vi "MultiTool-Track-Generate-ndipolarisFileOutput-Q-vectors-Accepts Joystick Command with Time Display-Improved PC clock in tcp loop.vi"() -> ()   [LabVIEW 2013]
panel:
  out "TIME":string
  out "bytes written":i32
  out "Return time string":string
  out "Length":u8
  out "Command":u8
  out "Tool 2":T1={"Port Handle"="", "Frame Number"=0, "Tx"=0.0, "Ty"=0.0, "Tz"=0.0, "Q0"=0.0, "Qx"=0.0, "Qy"=0.0, "Qz"=0.0, "Deviation"=0.0, " Markers Missing"=TRUE, "Out of Volume"=TRUE} {"Deviation" format="%#.4f"; "Qz" format="%#.4f"; "Qy" format="%#.4f"; "Qx" format="%#.4f"; "Q0" format="%#.4f"; "Tz" format="%#.2f"; "Ty" format="%#.2f"; "Tx" format="%#.2f"}
  in  "Location of ROM File for Tool 2":path=path "C:/Program Files (x86)/Northern Digital Inc/8700339.rom"
  in  "NDI  Running":bool=TRUE
  out "Stop Reading":bool=TRUE
  out "Start Reading":bool
  out "Object Identifier":string="0"
  in  "Track Outside Measurement Volume? (F:No)":bool
  in  "Track Stray Markers? (F:No)":bool
  out "Tool 1":T1={"Port Handle"="", "Frame Number"=0, "Tx"=0.0, "Ty"=0.0, "Tz"=0.0, "Q0"=0.0, "Qx"=0.0, "Qy"=0.0, "Qz"=0.0, "Deviation"=0.0, " Markers Missing"=TRUE, "Out of Volume"=TRUE} {"Deviation" format="%#.4f"; "Qz" format="%#.4f"; "Qy" format="%#.4f"; "Qx" format="%#.4f"; "Q0" format="%#.4f"; "Tz" format="%#.2f"; "Ty" format="%#.2f"; "Tx" format="%#.2f"}
  out "TCP loop":i32
  in  "TCP Server Running":bool=TRUE
  in  "Output Directory":path=path "C:/Users/Diogo/Desktop/NDI-Labview Gripper"
  out "NDI Loop":i32
  in  "VISA resource name":refnum<visa-resource-name>="COM8"
  in  "Reset? (T:Yes)":bool=TRUE
  in  "Location of ROM File for Tool 1":path=path "C:/Program Files (x86)/Northern Digital Inc/8700449.rom"
  in  "Serial Configuration":T2={"Baud Rate (9600)"=9600, "Flow Control (0:None)"=0, "Parity"=0, "Data Bits"=8, "Stop Bits"=10} {"Stop Bits" items=["1.0"=10, "2.0"=20]; "Parity" items=["None", "Odd", "Even"]; "Flow Control (0:None)" items=["None", "XON/XOFF"]; "Baud Rate (9600)" items=["9600"=9600, "14.4k"=14400, "19.2k"=19200, "38.4k"=38400, "57.6k "=57600, "115.2k"=115200]}
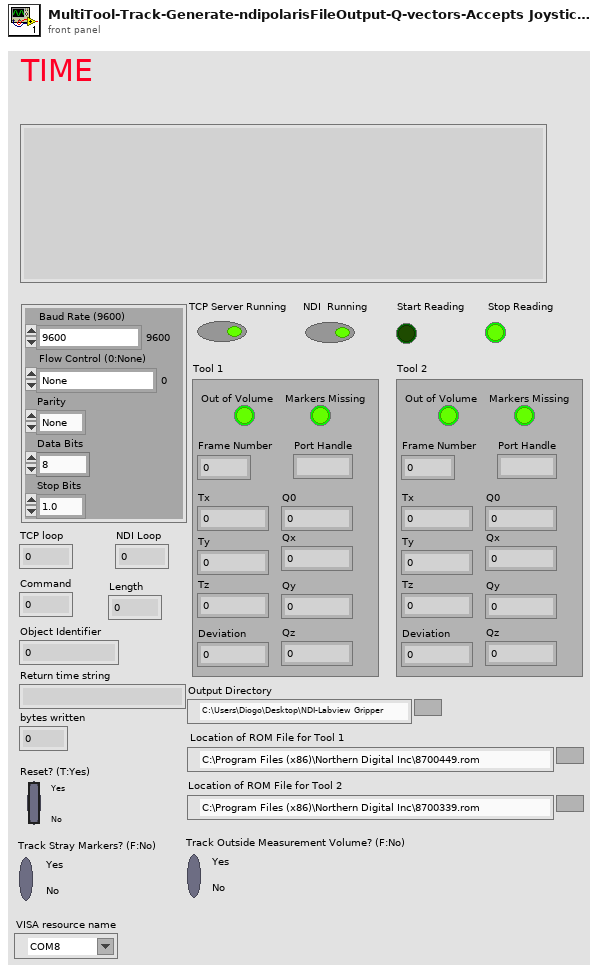
[diagram p1: front panel]
types:
  T1 = cluster{"Port Handle":string, "Frame Number":i32, "Tx":dbl, "Ty":dbl, "Tz":dbl, "Q0":dbl, "Qx":dbl, "Qy":dbl, "Qz":dbl, "Deviation":dbl, " Markers Missing":bool, "Out of Volume":bool}
  T2 = cluster{"Baud Rate (9600)":u32, "Flow Control (0:None)":u16, "Parity":u16, "Data Bits":u16, "Stop Bits":u16}
  T3 = cluster{"Port Handle":string, "Frame Number":u32, "Tx":dbl, "Ty":dbl, "Tz":dbl, "Q0":dbl, "Qx":dbl, "Qy":dbl, "Qz":dbl, "Deviation":dbl, "Missing?":bool, "Out of Volume?":bool}[]
  T4 = cluster{"Transformations[0]":cluster{"Port Handle":string, "Frame Number":u32, "Tx":dbl, "Ty":dbl, "Tz":dbl, "Q0":dbl, "Qx":dbl, "Qy":dbl, "Qz":dbl, "Deviation":dbl, "Missing?":bool, "Out of Volume?":bool}, "Transformations[1]":cluster{"Port Handle":string, "Frame Number":u32, "Tx":dbl, "Ty":dbl, "Tz":dbl, "Q0":dbl, "Qx":dbl, "Qy":dbl, "Qz":dbl, "Deviation":dbl, "Missing?":bool, "Out of Volume?":bool}, "Transformations[2]":cluster{"Port Handle":string, "Frame Number":u32, "Tx":dbl, "Ty":dbl, "Tz":dbl, "Q0":dbl, "Qx":dbl, "Qy":dbl, "Qz":dbl, "Deviation":dbl, "Missing?":bool, "Out of Volume?":bool}, "Transformations[3]":cluster{"Port Handle":string, "Frame Number":u32, "Tx":dbl, "Ty":dbl, "Tz":dbl, "Q0":dbl, "Qx":dbl, "Qy":dbl, "Qz":dbl, "Deviation":dbl, "Missing?":bool, "Out of Volume?":bool}, "Transformations[4]":cluster{"Port Handle":string, "Frame Number":u32, "Tx":dbl, "Ty":dbl, "Tz":dbl, "Q0":dbl, "Qx":dbl, "Qy":dbl, "Qz":dbl, "Deviation":dbl, "Missing?":bool, "Out of Volume?":bool}, "Transformations[5]":cluster{"Port Handle":string, "Frame Number":u32, "Tx":dbl, "Ty":dbl, "Tz":dbl, "Q0":dbl, "Qx":dbl, "Qy":dbl, "Qz":dbl, "Deviation":dbl, "Missing?":bool, "Out of Volume?":bool}, "Transformations[6]":cluster{"Port Handle":string, "Frame Number":u32, "Tx":dbl, "Ty":dbl, "Tz":dbl, "Q0":dbl, "Qx":dbl, "Qy":dbl, "Qz":dbl, "Deviation":dbl, "Missing?":bool, "Out of Volume?":bool}, "Transformations[7]":cluster{"Port Handle":string, "Frame Number":u32, "Tx":dbl, "Ty":dbl, "Tz":dbl, "Q0":dbl, "Qx":dbl, "Qy":dbl, "Qz":dbl, "Deviation":dbl, "Missing?":bool, "Out of Volume?":bool}, "Transformations[8]":cluster{"Port Handle":string, "Frame Number":u32, "Tx":dbl, "Ty":dbl, "Tz":dbl, "Q0":dbl, "Qx":dbl, "Qy":dbl, "Qz":dbl, "Deviation":dbl, "Missing?":bool, "Out of Volume?":bool}}
  T5 = cluster{"Port Handle":string, "Frame Number":u32, "Tx":dbl, "Ty":dbl, "Tz":dbl, "Q0":dbl, "Qx":dbl, "Qy":dbl, "Qz":dbl, "Deviation":dbl, "Missing?":bool, "Out of Volume?":bool}
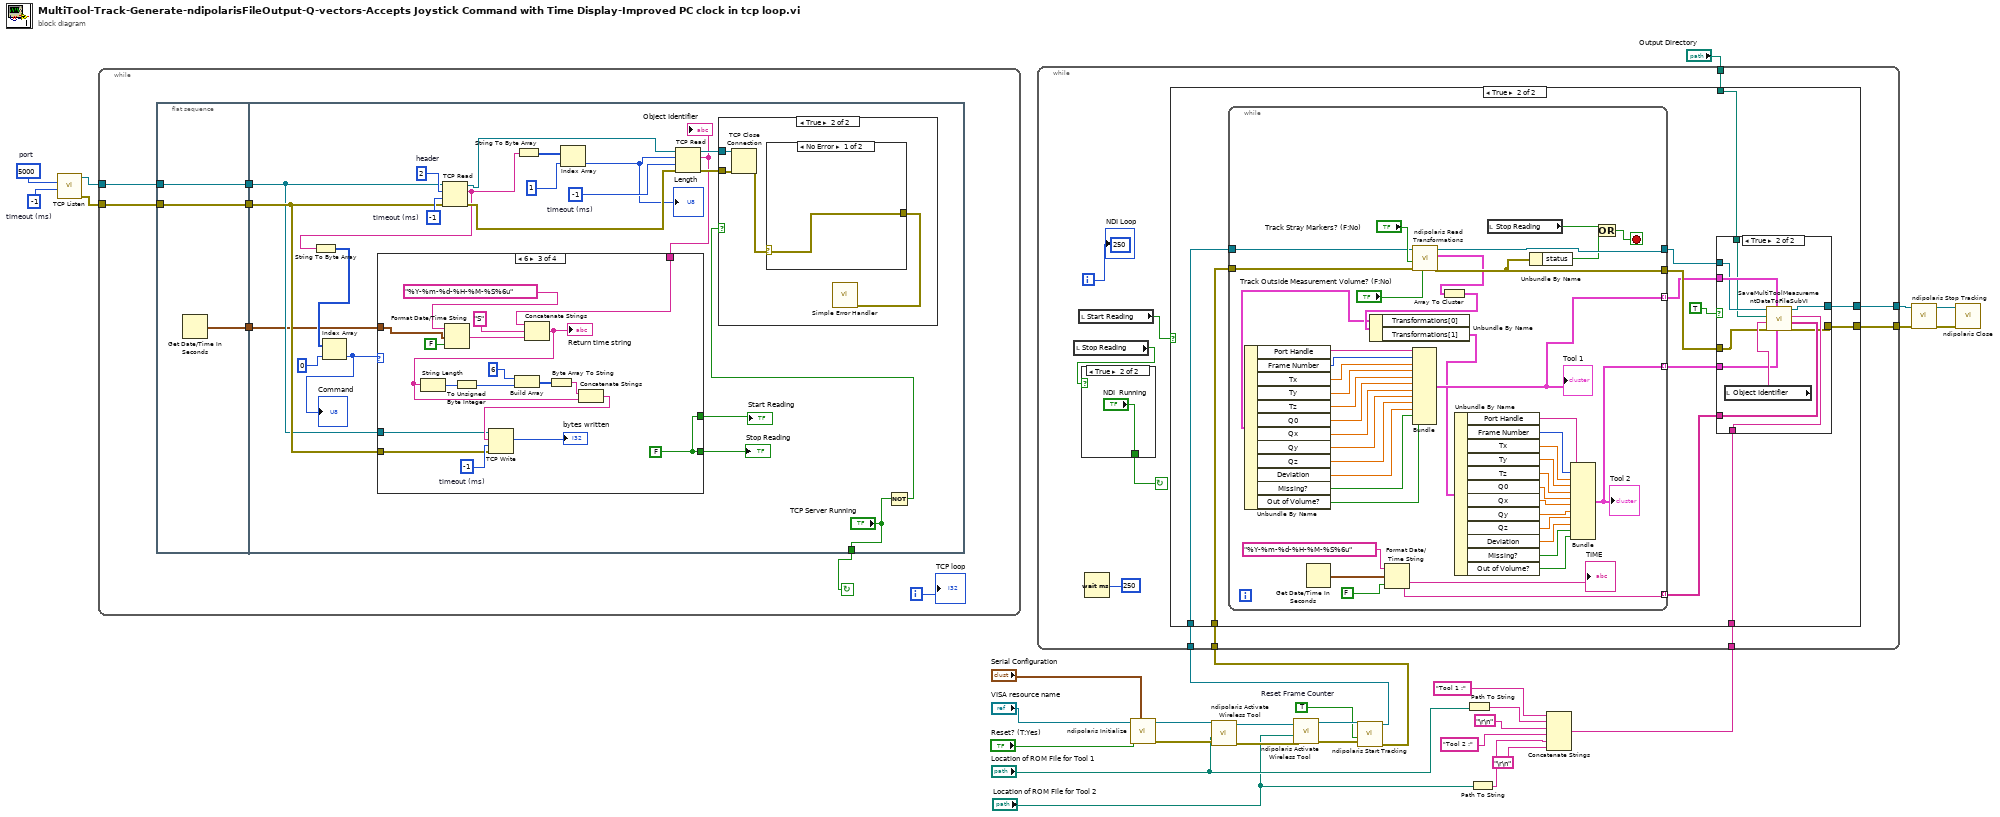
[diagram p0: block diagram]
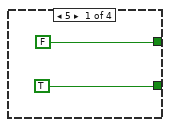
[diagram p2: hidden frame]
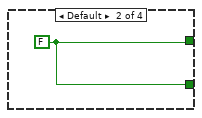
[diagram p3: hidden frame]
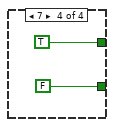
[diagram p4: hidden frame]
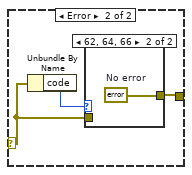
[diagram p6: hidden frame]
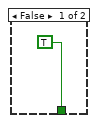
[diagram p8: hidden frame]
diagram:
  w21 = TRUE  # Reset Frame Counter
  w30 = u16 5000  # port
  w29 = i8 -1  # timeout (ms)
  n1 = call <vilib>:"TCP Listen.vi"("timeout ms (wait forever: -1)"=w29, "port"=w30) -> ("error out"=w24:errorcluster, "connection ID"=w25:refnum<k5>)  [unwired: 5 in, 3 out]
  n2 = while {
    tunnel: w25 -> [w34]
    tunnel: w24 -> [w35]
    i -> [w37]
    stop <- w36 continue-if-true
    n3 = flat-sequence {
      tunnel: w34 -> [w39]
      tunnel: w35 -> [w40]
      tunnel: [w40] -> w33
      tunnel: [w39] -> w32
      tunnel: [w38] -> w31
      tunnel: ["TCP Server Running"] -> w36
      tunnel: w33 -> [w44]
      tunnel: w32 -> [w42]
      tunnel: w31 -> [w41]
      frame #0 {
        n4 = Get Date/Time In Seconds() -> (seconds since 1Jan1904=w38:timestamp)
      }
      frame #1 {
        w58 = i8 -1  # timeout (ms)
        w61 = i8 -1  # timeout (ms)
        w62 = i8 2  # header
        n5 = TCP Read(connection ID=w42, bytes to read=w62, error in (no error)=w44, 9:w61) -> (connection ID out=w60:refnum<k5>, data out=w49:string, error out=w59:errorcluster)  [unwired: 1 in]
        n6 = String To Byte Array(string=w49) -> (unsigned byte array=w52:u8[])
        n7 = Index Array(array=w52, index=0) -> (element=w45:u8)
        "Command" <- w45
        n8 = String To Byte Array(string=w49) -> (unsigned byte array=w51:u8[])
        n9 = Index Array(array=w51, index=1) -> (element=w48:u8)
        "Length" <- w48
        n10 = TCP Read(connection ID=w60, bytes to read=w48, error in (no error)=w59, 9:w58) -> (connection ID out=w57:refnum<k5>, data out=w43:string, error out=w56:errorcluster)  [unwired: 1 in]
        "Object Identifier" <- w43
        n11 = case shown="6" w45 {
          tunnel: [FALSE w65 w67 TRUE] -> w55
          tunnel: [TRUE w65 w67 FALSE] -> w54
          tunnel: w44 -> [_ _ w70 _]
          tunnel: w43 -> [_ _ w69 _]
          tunnel: w42 -> [_ _ w68 _]
          tunnel: w41 -> [_ _ w66 _]
          frame 5 {
          }
          frame Default {
            w65 = FALSE
          }
          frame 6 {
            w79 = i8 -1  # timeout (ms)
            w67 = FALSE
            n12 = Format Date/Time String(time format string (%c)="%Y-%m-%d-%H-%M-%S%6u", seconds (now)=w66, UTC format=FALSE) -> (date/time string=w83:string)
            n13 = Concatenate Strings(w69, "S", w83) -> (w72:string)
            "Return time string" <- w72
            n14 = String Length(string=w72) -> (length=w76:i32)
            n15 = To Unsigned Byte Integer(number=w76) -> (unsigned 8bit integer=w75:u8)
            n16 = Build Array(u8 6, w75) -> (w73:u8[])
            n17 = Byte Array To String(unsigned byte array=w73) -> (string=w78:string)
            n18 = Concatenate Strings(w78, w72) -> (w71:string)
            n19 = TCP Write(connection ID=w68, data in=w71, error in (no error)=w70, 9:w79) -> (bytes written=→"bytes written":i32)  [unwired: 2 out]
          }
          frame 7 {
          }
        }
        "Start Reading" <- w55
        "Stop Reading" <- w54
        n20 = Not(x="TCP Server Running") -> (.not. x?=w46:bool)
        n21 = case shown="True" w46 {
          tunnel: w57 -> [_ w87]
          tunnel: w56 -> [_ w86]
          frame False {
          }
          frame True {
            n22 = TCP Close Connection(connection ID=w87, error in (no error)=w86) -> (error out=w88:errorcluster)  [unwired: 1 in, 1 out]
            n23 = case shown="No Error" w88 {
              selector: w88 -> [w90 w92]
              tunnel: [w90 w91] -> w89
              frame No Error {
              }
              frame Error {
                n24 = Unbundle By Name(w92) -> ("code"=w93:i32)
                n25 = case shown="62, 64, 66" w93 {
                  tunnel: w92 -> [w94 _]
                  tunnel: [w94 w95] -> w91
                  frame Default {
                  }
                  frame 62, 64, 66 {
                    w95 = errorcluster {"status"=FALSE, "code"=0, "source"=""}  # No error
                  }
                }
              }
            }
            n26 = call <vilib>:"Simple Error Handler.vi"("error in (no error)"=w89) -> ()  [unwired: 1 in, 8 out]
          }
        }
      }
    }
    "TCP loop" <- w37
  }
  n27 = call <instrlib>:"ndipolaris Initialize.vi"("Serial Configuration"="Serial Configuration", "Reset? (T: Yes)"="Reset? (T:Yes)", "VISA resource name"="VISA resource name") -> ("error out"=w11:errorcluster, "VISA resource name out"=w12:refnum<visa-resource-name>)  [unwired: 7 in]
  n28 = call <instrlib>:"ndipolaris Activate Wireless Tool.vi"("error in (no error)"=w11, "Location of ROM File for Tool"="Location of ROM File for Tool 1", "VISA resource name"=w12) -> ("error out"=w9:errorcluster, "VISA resource out"=w10:refnum<visa-resource-name>)  [unwired: 6 in, 1 out]
  n29 = call <instrlib>:"ndipolaris Activate Wireless Tool.vi"("error in (no error)"=w9, "Location of ROM File for Tool"="Location of ROM File for Tool 2", "VISA resource name"=w10) -> ("error out"=w22:errorcluster, "VISA resource out"=w23:refnum<visa-resource-name>)  [unwired: 6 in, 1 out]
  n30 = call <instrlib>:"ndipolaris Start Tracking.vi"("error in (no error)"=w22, "Reset Frame Counter? (F:No)"=w21, "VISA resource name"=w23) -> ("error out"=w16:errorcluster, "VISA resource out"=w20:refnum<visa-resource-name>)  [unwired: 7 in]
  n31 = Path To String(path="Location of ROM File for Tool 1") -> (string=w5:string)
  n32 = Path To String(path="Location of ROM File for Tool 2") -> (string=w3:string)
  n33 = Concatenate Strings("Tool 1 :" ("string"), w5, "\r\n", "Tool 2 :" ("string"), w3, "\r\n") -> (w13:string)
  n34 = while {
    tunnel: w20 -> [w105]
    tunnel: [w104] -> w17
    tunnel: w16 -> [w103]
    tunnel: "Output Directory" -> [w102]
    tunnel: [w101] -> w14
    tunnel: w13 -> [w97]
    i -> [w106]
    stop <- w96 continue-if-true
    (unwired) u8 250
    n35 = local read "Stop Reading"() -> (w98:bool)
    n36 = local read "Start Reading"() -> (w99:bool)
    n37 = case shown="True" w98 {
      tunnel: [TRUE "NDI  Running"] -> w96
      frame False {
      }
      frame True {
      }
    }
    n38 = Wait (ms)(milliseconds to wait=u32 250) -> ()  [unwired: 1 out]
    n39 = case shown="True" w99 {
      tunnel: w105 -> [w110 w122]
      tunnel: [w110 w118] -> w104
      tunnel: w103 -> [w109 w121]
      tunnel: w102 -> [_ w120]
      tunnel: [w109 w117] -> w101
      tunnel: w97 -> [_ w112]
      frame False {
      }
      frame True {
        n40 = while {
          tunnel: [w176] -> w114
          tunnel: [w175] -> w119
          tunnel: [w152] -> w115 mode=indexing
          tunnel: [w153] -> w116 mode=indexing
          tunnel: w122 -> [w151]
          tunnel: w121 -> [w150]
          tunnel: [w135] -> w111 mode=indexing
          stop <- w177 stop-if-true
          n41 = Get Date/Time In Seconds() -> (seconds since 1Jan1904=w156:timestamp)
          n42 = Format Date/Time String(time format string (%c)="%Y-%m-%d-%H-%M-%S%6u", seconds (now)=w156, UTC format=FALSE) -> (date/time string=w153:string)
          "TIME" <- w153
          n43 = call <instrlib>:"ndipolaris Read Transformations.vi"("Track Outside Measurement Volume? (F:No)"="Track Outside Measurement Volume? (F:No)", "error in (no error)"=w150, "Track Stray Markers? (F:No)"="Track Stray Markers? (F:No)", "VISA resource name"=w151) -> ("error out"=w175:errorcluster, "Transformations"=w160:T3, "VISA resource out"=w176:refnum<visa-resource-name>)  [unwired: 4 in, 1 out]
          n44 = Array To Cluster(array=w160) -> (cluster=w171:T4)
          n45 = Unbundle By Name(w171) -> ("Transformations[0]"=w170:T5, "Transformations[1]"=w148:T5)
          n46 = Unbundle By Name(w170) -> ("Port Handle"=w169:string, "Frame Number"=w168:u32, "Tx"=w167:dbl, "Ty"=w166:dbl, "Tz"=w165:dbl, "Q0"=w164:dbl, "Qx"=w163:dbl, "Qy"=w162:dbl, "Qz"=w161:dbl, "Deviation"=w159:dbl, "Missing?"=w158:bool, "Out of Volume?"=w157:bool)
          n47 = Bundle("Port Handle"=w169, "Frame Number"=w168, "Tx"=w167, "Ty"=w166, "Tz"=w165, "Q0"=w164, "Qx"=w163, "Qy"=w162, "Qz"=w161, "Deviation"=w159, "Missing?"=w158, "Out of Volume?"=w157) -> (w152:T5)  [unwired: 1 in]
          "Tool 1" <- w152
          n48 = Unbundle By Name(w148) -> ("Port Handle"=w147:string, "Frame Number"=w146:u32, "Tx"=w145:dbl, "Ty"=w144:dbl, "Tz"=w143:dbl, "Q0"=w142:dbl, "Qx"=w141:dbl, "Qy"=w140:dbl, "Qz"=w139:dbl, "Deviation"=w138:dbl, "Missing?"=w137:bool, "Out of Volume?"=w136:bool)
          n49 = local read "Stop Reading"() -> (w149:bool)
          n50 = Unbundle By Name(w175) -> ("status"=w174:bool)
          n51 = Bundle("Port Handle"=w147, "Frame Number"=w146, "Tx"=w145, "Ty"=w144, "Tz"=w143, "Q0"=w142, "Qx"=w141, "Qy"=w140, "Qz"=w139, "Deviation"=w138, "Missing?"=w137, "Out of Volume?"=w136) -> (w135:T5)  [unwired: 1 in]
          "Tool 2" <- w135
          n52 = Or(x=w149, y=w174) -> (x .or. y?=w177:bool)
        }
        n53 = case shown="True" TRUE {
          tunnel: w120 -> [_ w132]
          tunnel: w119 -> [w123 w130]
          tunnel: [w124 w129] -> w118
          tunnel: [w123 w125] -> w117
          tunnel: w116 -> [_ w128]
          tunnel: w115 -> [_ w134]
          tunnel: w114 -> [w124 w133]
          tunnel: w112 -> [_ w127]
          tunnel: w111 -> [_ w126]
          frame False {
          }
          frame True {
            n54 = local read "Object Identifier"() -> (w131:string)
            n55 = call "SaveMultiToolMeasurementDataToFileSubVI.vi"("Array of Time for Measurement"=w128, "NDI Tool"=w127, "Array - Transformations of Tool 2"=w126, "Array - Transformations of Tool 1"=w134, "error in (no error)"=w130, "Object number"=w131, "Output Directory"=w132, "VISA Refnum in"=w133) -> ("error out"=w125:errorcluster, "VISA Refnum out"=w129:refnum<visa-resource-name>)
          }
        }
      }
    }
    "NDI Loop" <- w106
  }
  n56 = call <instrlib>:"ndipolaris Stop Tracking.vi"("error in (no error)"=w14, "VISA resource name"=w17) -> ("error out"=w18:errorcluster, "VISA resource out"=w19:refnum<visa-resource-name>)  [unwired: 8 in]
  n57 = call <instrlib>:"ndipolaris Close.vi"("error in (no error)"=w18, "VISA resource name"=w19) -> ()  [unwired: 9 in, 1 out]
